vi "Sync B-Scan Demo.vi"() -> ()   [LabVIEW 2012]
uses:
  LabVIEW/user.lib/SpectralRadar.llb/set Scan Output.vi
  LabVIEW/user.lib/SpectralRadar.llb/set Spectrum Output.vi
  LabVIEW/user.lib/SpectralRadar.llb/display Data 2D.vi
  LabVIEW/user.lib/SpectralRadar.llb/OCT Device.lvclass
  LabVIEW/user.lib/SpectralRadar.llb/Probe.lvclass
  LabVIEW/user.lib/SpectralRadar.llb/Processing.lvclass
  LabVIEW/user.lib/SpectralRadar.llb/Scan Pattern.lvclass
  LabVIEW/user.lib/SpectralRadar.llb/Raw Data.lvclass
  LabVIEW/user.lib/SpectralRadar.llb/Data.lvclass
panel:
  in  "stop":bool
  out "B-Scan Data":dbl[][](graph)
  out "Spectral Data":dbl[][](graph)
  in  "AScans":i32=512
  in  "Range [mm]":dbl=2.0 min=0.0 format="%_4f"
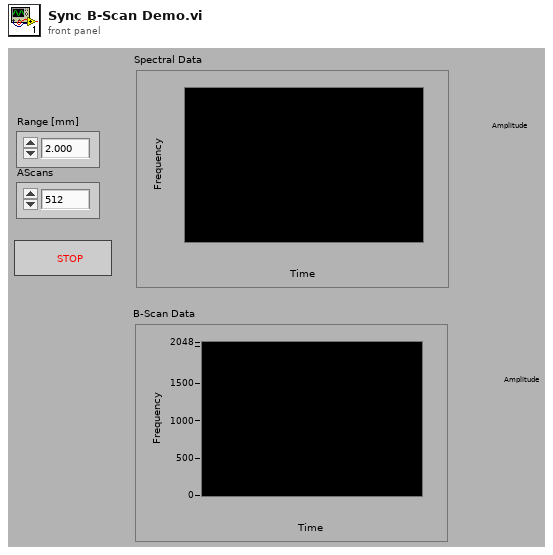
[diagram p1: front panel]
types:
  T1 = enum16{"Asynchronous Continuous", "Asynchronous Finite", "Synchronous"}
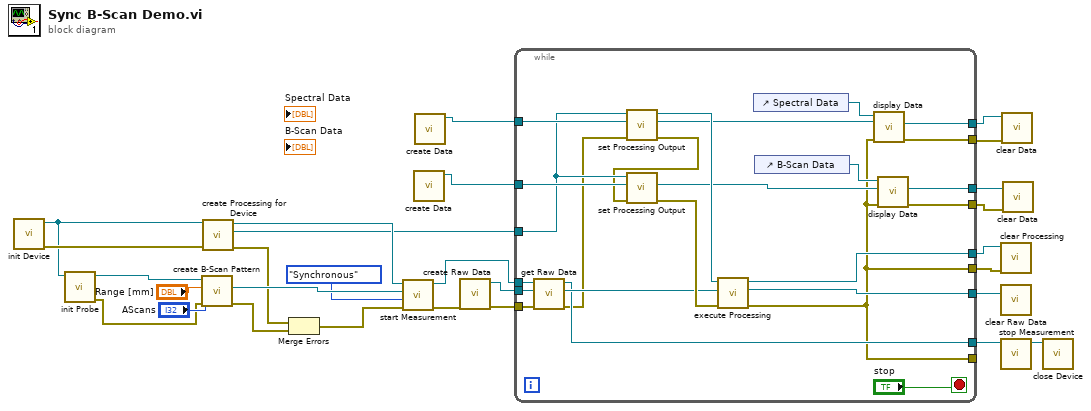
[diagram p0: block diagram]
diagram:
  n1 = call "init Device.vi"() -> ("error out"=w28:errorcluster, "OCTDevice"=w13:refnum<class "OCT Device.lvclass">)  [unwired: 6 in]
  n2 = call "init Probe.vi"("OCT Device"=w13) -> ("error out"=w12:errorcluster, "GalvoControl"=w27:refnum<class "Probe.lvclass">)  [unwired: 5 in]
  n3 = call "create B-Scan Pattern.vi"("error in (no error)"=w12, "AScans"="AScans", "Range"="Range [mm]", "Probe"=w27) -> ("error out"=w22:errorcluster, "Scan Pattern"=w24:refnum<class "Scan Pattern.lvclass">)  [unwired: 2 in, 1 out]
  n4 = call "create Processing for Device.vi"("error in (no error)"=w28, "OCTDevice"=w13) -> ("error out"=w20:errorcluster, "Processing"=w15:refnum<class "Processing.lvclass">, "OCTDevice"=w16:refnum<class "OCT Device.lvclass">)  [unwired: 3 in]
  n5 = Merge Errors(w20, w22) -> (w21:errorcluster)
  n6 = call "start Measurement.vi"("error in (no error)"=w21, "Acquisition Type"=T1."Synchronous", "Scan Pattern"=w24, "OCTDevice"=w16) -> ("error out"=w18:errorcluster, "OCTDevice"=w9:refnum<class "OCT Device.lvclass">)  [unwired: 1 in, 1 out]
  n7 = call "create Data.vi"() -> ("Data"=w8:refnum<class "Data.lvclass">)  [unwired: 6 in, 1 out]
  n8 = call "create Data.vi"() -> ("Data"=w7:refnum<class "Data.lvclass">)  [unwired: 6 in, 1 out]
  n9 = call "create Raw Data.vi"("error in (no error)"=w18) -> ("error out"=w17:errorcluster, "Raw Data"=w19:refnum<class "Raw Data.lvclass">)  [unwired: 5 in]
  n10 = while {
    tunnel: w19 -> [w51]
    tunnel: w9 -> [w52]
    tunnel: w17 -> [w50]
    tunnel: w15 -> [w47]
    tunnel: w8 -> [w49]
    tunnel: w7 -> [w48]
    tunnel: [w38] -> w14
    tunnel: [w37] -> w2
    tunnel: [w36] -> w4
    tunnel: [w35] -> w6
    tunnel: [w34] -> w3
    tunnel: [w33] -> w5
    tunnel: [w32] -> w11
    tunnel: [w30] -> w1
    tunnel: [w30] -> _
    stop <- "stop" stop-if-true
    n11 = call "get Raw Data.vi"("error in (no error)"=w50, "RawData in"=w51, "OCTDevice in"=w52) -> ("error out"=w31:errorcluster, "RawData out"=w43:refnum<class "Raw Data.lvclass">, "OCTDevice out"=w32:refnum<class "OCT Device.lvclass">)  [unwired: 2 in]
    n12 = call-poly "set Processing Output.vi"("error in (no error)"=w31, "Data"=w48, "Processing"=w47) -> ("error out"=w45:errorcluster, "Data"=w41:refnum<class "Data.lvclass">, "Processing"=w46:refnum<class "Processing.lvclass">)  [unwired: 2 in]
    n13 = call-poly "set Processing Output.vi"("error in (no error)"=w45, "Data"=w49, "Processing"=w47) -> ("error out"=w44:errorcluster, "Data"=w39:refnum<class "Data.lvclass">)  [unwired: 2 in, 1 out]
    n14 = call "execute Processing.vi"("error in (no error)"=w44, "Raw Data"=w43, "Processing"=w46) -> ("error out"=w30:errorcluster, "Raw Data"=w38:refnum<class "Raw Data.lvclass">, "Processing"=w37:refnum<class "Processing.lvclass">)  [unwired: 2 in]
    n15 = control-ref of="Spectral Data"() -> (w42:refnum<vi>)
    n16 = control-ref of="B-Scan Data"() -> (w40:refnum<vi>)
    n17 = call-poly "display Data.vi"("error in (no error)"=w30, "Data in"=w41, "IntGraph Refnum"=w42) -> ("error out"=w33:errorcluster, "Data out"=w35:refnum<class "Data.lvclass">)  [unwired: 2 in, 1 out]
    n18 = call-poly "display Data.vi"("error in (no error)"=w30, "Data in"=w39, "IntGraph Refnum"=w40) -> ("error out"=w34:errorcluster, "Data out"=w36:refnum<class "Data.lvclass">)  [unwired: 2 in, 1 out]
  }
  n19 = call "clear Processing.vi"("error in (no error)"=w1, "Processing"=w2) -> ()  [unwired: 5 in, 1 out]
  n20 = call "clear Raw Data.vi"("Raw Data"=w14) -> ()  [unwired: 6 in, 1 out]
  n21 = call "stop Measurement.vi"("OCTDevice"=w11) -> ("OCTDevice"=w10:refnum<class "OCT Device.lvclass">)  [unwired: 5 in, 1 out]
  n22 = call "clear Data.vi"("error in (no error)"=w5, "Data"=w6) -> ()  [unwired: 5 in, 1 out]
  n23 = call "clear Data.vi"("error in (no error)"=w3, "Data"=w4) -> ()  [unwired: 5 in, 1 out]
  n24 = call "close Device.vi"("OCTDevice"=w10) -> ()  [unwired: 6 in, 1 out]
